vi "In Place Element Structure - Map Border Nodes.vi"   [LabVIEW 2020]
doc: "Places an In Place Element structure on the block diagram with the Map Get / Replace Value border node added."
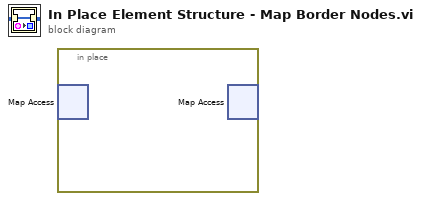
[diagram p0: block diagram]
diagram:
  n1 = in-place {
    n2 = in-place-map #1() -> ()  [unwired: 3 in, 2 out]
    n3 = in-place-map #1() -> ()  [unwired: 2 in, 3 out]
  }
